vi "Write.vi"(8 "error in (no error)":errorcluster, 11 "Hardware Resources in":T1) -> (0 "error out":errorcluster, 3 "Hardware Resources out":T1)   [LabVIEW 2018, in "DAQ.lvlib"]
doc: "Perform the acquisition. Replace the contents of this diagram with calls to acquisition hardware."
uses:
  DAQ/DAQ.lvlib
  <resource>/objmgr/daqmx.rc
  <vilib>/DAQmx/write.llb/DAQmx Write (Digital 1D Bool NChan 1Samp 1Line).vi
  Hardware Configuration.ctl
  Task Cluster.ctl
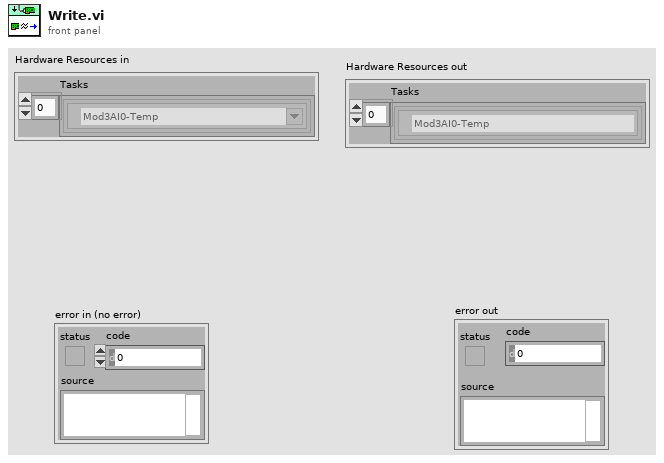
[diagram p1: front panel]
types:
  T1 = typedef "DAQ.lvlib/Hardware Configuration.ctl" = cluster{"Tasks":T2[]}
  T2 = typedef "Task Cluster.ctl" = cluster{"DAQmx Task":refnum<k21>}
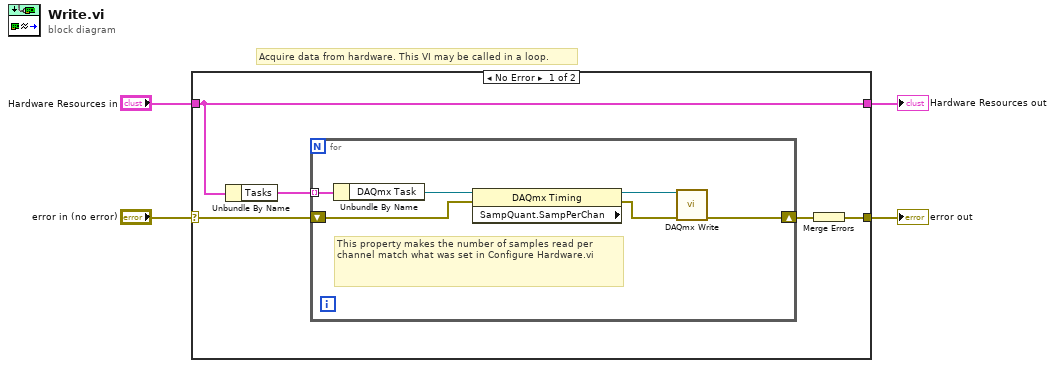
[diagram p0: block diagram]
diagram:
  # "Acquire data from hardware. This VI may be called in a loop."
  n1 = case shown="No Error" "error in (no error)" {
    selector: "error in (no error)" -> [w5 w16]
    tunnel: [w9 w16] -> w3
    tunnel: "Hardware Resources in" -> [w8 w17]
    tunnel: [w8 w17] -> w1
    frame No Error {
      n2 = Unbundle By Name(w8) -> ("Tasks"=w6:T2[])
      n3 = for {
        tunnel: w6 -> [w14] mode=indexing
        shift-right: [w15] -> w7
        shift-left: w5 -> [w12]
        # "This property makes the number of samples read per channel match what was set in Configure Hardware.vi"
        n4 = Unbundle By Name(w14) -> ("DAQmx Task"=w10:refnum<k21>)
        n5 = property class="DAQmx Timing" props=["SampQuant.SampPerChan"](reference=w10, error in=w12) -> (reference out=w13:refnum<k21>, error out=w11:errorcluster)  [unwired: 1 out]
        n6 = call-poly <vilib>:"DAQmx Write.vi"("task/channels in"=w13, "error in"=w11) -> ("error out"=w15:errorcluster)  [unwired: 11 in, 2 out]
      }
      n7 = Merge Errors(w7) -> (w9:errorcluster)
    }
    frame Error {
    }
  }
  "Hardware Resources out" <- w1
  "error out" <- w3
